vi "Path - When Not Constructed - Is Empty.vi"() -> ()   [LabVIEW 2017, in "Test Case.Tests.lvlib"]
uses:
  Test Case.Tests.lvlib
  Test Case/Test Case.lvclass
  Test Case/Test Case.lvclass/Test Case.ctl
  fc41dd10-c4f1-4a55-a86a-822b6e90fa10.vi
  Test Case/Get Path.vi
  Constraint/IsEqual/Create.vi
  Constraint/IsEqual/IsEqual.lvclass
panel:
  out "error out":errorcluster
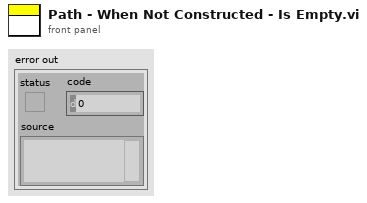
[diagram p1: front panel]
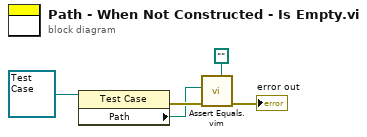
[diagram p0: block diagram]
diagram:
  n1 = property class="Test Case"(reference=refnum<class "Test Case.lvclass"> refnum ("Test Case")) -> (error out=w4:errorcluster, "Path"=w3:path)  [unwired: 1 in, 1 out]
  n2 = call "Assert Equals.vim"("Expected"=path "" ("Path"), "error in (no error)"=w4, "Actual"=w3) -> ("error out"=→"error out":errorcluster)  [unwired: 8 in]
